vi "Read Collected Data.vi"(8 "error in (no error)":errorcluster, 11 "AbstractCollector in":refnum<class "AbstractCollector.lvclass">) -> (0 "error out":errorcluster, 2 "Collected Data":refnum<class "AbstractData.lvclass">, 3 "AbstractCollector out":refnum<class "AbstractCollector.lvclass">)   [LabVIEW 2014, in "AbstractCollector.lvclass"]
uses:
  AbstractCollector.lvclass
  Model/Data/AbstractData/AbstractData.lvclass
  AbstractCollector.lvclass/AbstractCollector.ctl
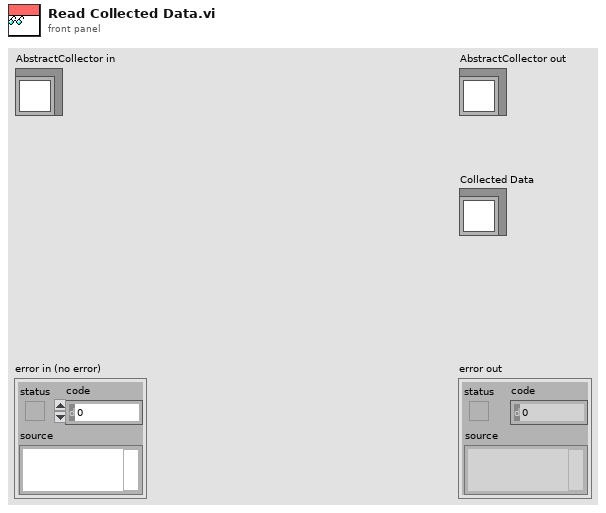
[diagram p1: front panel]
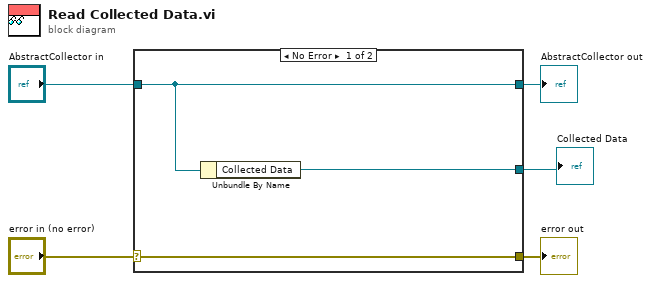
[diagram p0: block diagram]
diagram:
  n1 = case shown="No Error" "error in (no error)" {
    selector: "error in (no error)" -> [w8 w9]
    tunnel: [w8 w9] -> w4
    tunnel: [w7 w10] -> w2
    tunnel: "AbstractCollector in" -> [w7 w10]
    tunnel: [w6 _] -> w1
    frame No Error {
      n2 = Unbundle By Name(w7) -> ("Collected Data"=w6:refnum<class "AbstractData.lvclass">)
    }
    frame Error {
    }
  }
  "error out" <- w4
  "AbstractCollector out" <- w2
  "Collected Data" <- w1
